vi "Clockwise.vi"(10 "Count(Ticks)":u32 caption="计数器(滴答)") -> ()   [LabVIEW 2012]
uses:
  <vilib>/rvi/eio/common/nirviEmuTemplateMethod_errors.vi
  <vilib>/eio/EIONode/EIONode.xnode
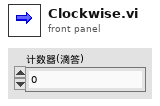
[diagram p1: front panel]
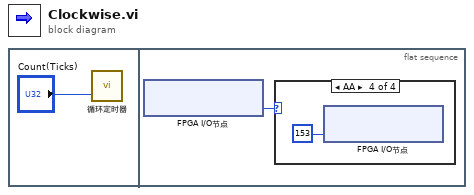
[diagram p0: block diagram]
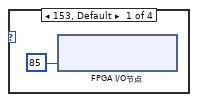
[diagram p2: hidden frame]
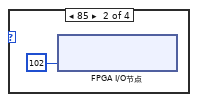
[diagram p3: hidden frame]
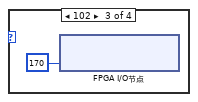
[diagram p4: hidden frame]
diagram:
  n1 = flat-sequence {
    frame #0 {
      n2 = call "循环定时器"("Count(Ticks)"="Count(Ticks)") -> ()  [unwired: 1 out]
    }
    frame #1 {
      n3 = xnode "FPGA I/O节点"() -> ("Port6/DIO9:0"=w2:u16)  [unwired: 1 in, 1 out]
      n4 = case shown="AA" w2 {
        frame 153, Default {
          n5 = xnode "FPGA I/O节点"("Port6/DIO9:0"=u16 85) -> ()  [unwired: 1 in, 1 out]
        }
        frame 85 {
          n6 = xnode "FPGA I/O节点"("Port6/DIO9:0"=u16 102) -> ()  [unwired: 1 in, 1 out]
        }
        frame 102 {
          n7 = xnode "FPGA I/O节点"("Port6/DIO9:0"=u16 170) -> ()  [unwired: 1 in, 1 out]
        }
        frame 170 {
          n8 = xnode "FPGA I/O节点"("Port6/DIO9:0"=u16 153) -> ()  [unwired: 1 in, 1 out]
        }
      }
    }
  }
